vi "DispatchService.vi"   [LabVIEW 2011]
uses:
  AnyService.dll
panel:
  # "No panel controls - see diagram"
types:
  T1 = typedef "Rendezvous RefNum" = refnum<k1>
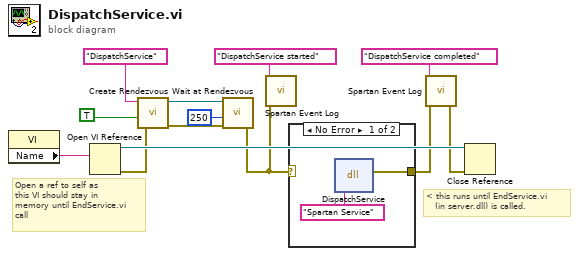
[diagram p0: block diagram]
diagram:
  # "Open a ref to self as\nthis VI should stay in\nmemory until EndService.vi\ncall"
  # "< this runs until EndService.vi\n   (in server.dll) is called."
  n1 = property class="VI"() -> ("Name"=w5:string)  [unwired: 2 in, 2 out]
  n2 = Open VI Reference(vi path=w5) -> (vi reference=w11:refnum<vi>, error out=w4:errorcluster)  [unwired: 5 in]
  n3 = call <vilib>:"Create Rendezvous.vi"("error in (no error)"=w4, "return existing (F)"=TRUE, "name (unnamed)"="DispatchService") -> ("error out"=w6:errorcluster, "rendezvous"=w7:T1)  [unwired: 2 in, 1 out]
  n4 = call <vilib>:"Wait at Rendezvous.vi"("error in (no error)"=w6, "ms timeout (-1)"=250, "rendezvous"=w7) -> ("error out"=w3:errorcluster)  [unwired: 2 in, 2 out]
  n5 = call "Spartan Event Log.vi"("error in (no error)"=w3, "message (\"\")"="DispatchService started") -> ()  [unwired: 6 in, 1 out]
  n6 = case shown="No Error" w3 {
    selector: w3 -> [_ w16]
    tunnel: [w15 w16] -> w1
    frame No Error {
      n7 = dll-call lib="C:/Development/Spartan/server/service/AnyService.dll" fn="DispatchService"("serviceName"="Spartan Service") -> (error out=w15:errorcluster)  [unwired: 3 in, 3 out]
    }
    frame Error {
    }
  }
  n8 = call "Spartan Event Log.vi"("error in (no error)"=w1, "message (\"\")"="DispatchService completed") -> ("error out"=w2:errorcluster)  [unwired: 6 in]
  n9 = Close Reference(reference=w11, error in (no error)=w2) -> ()  [unwired: 1 out]
